vi "vi for testing code.vi"() -> ()   [LabVIEW 2020]
panel:
  out "XY Graph":T1(graph)
  out "acc 3":dbl[](array[numeric])
  out "tt 2":dbl[](array[numeric])
  out "appended path":path
  out "array":dbl[][](array[numeric])
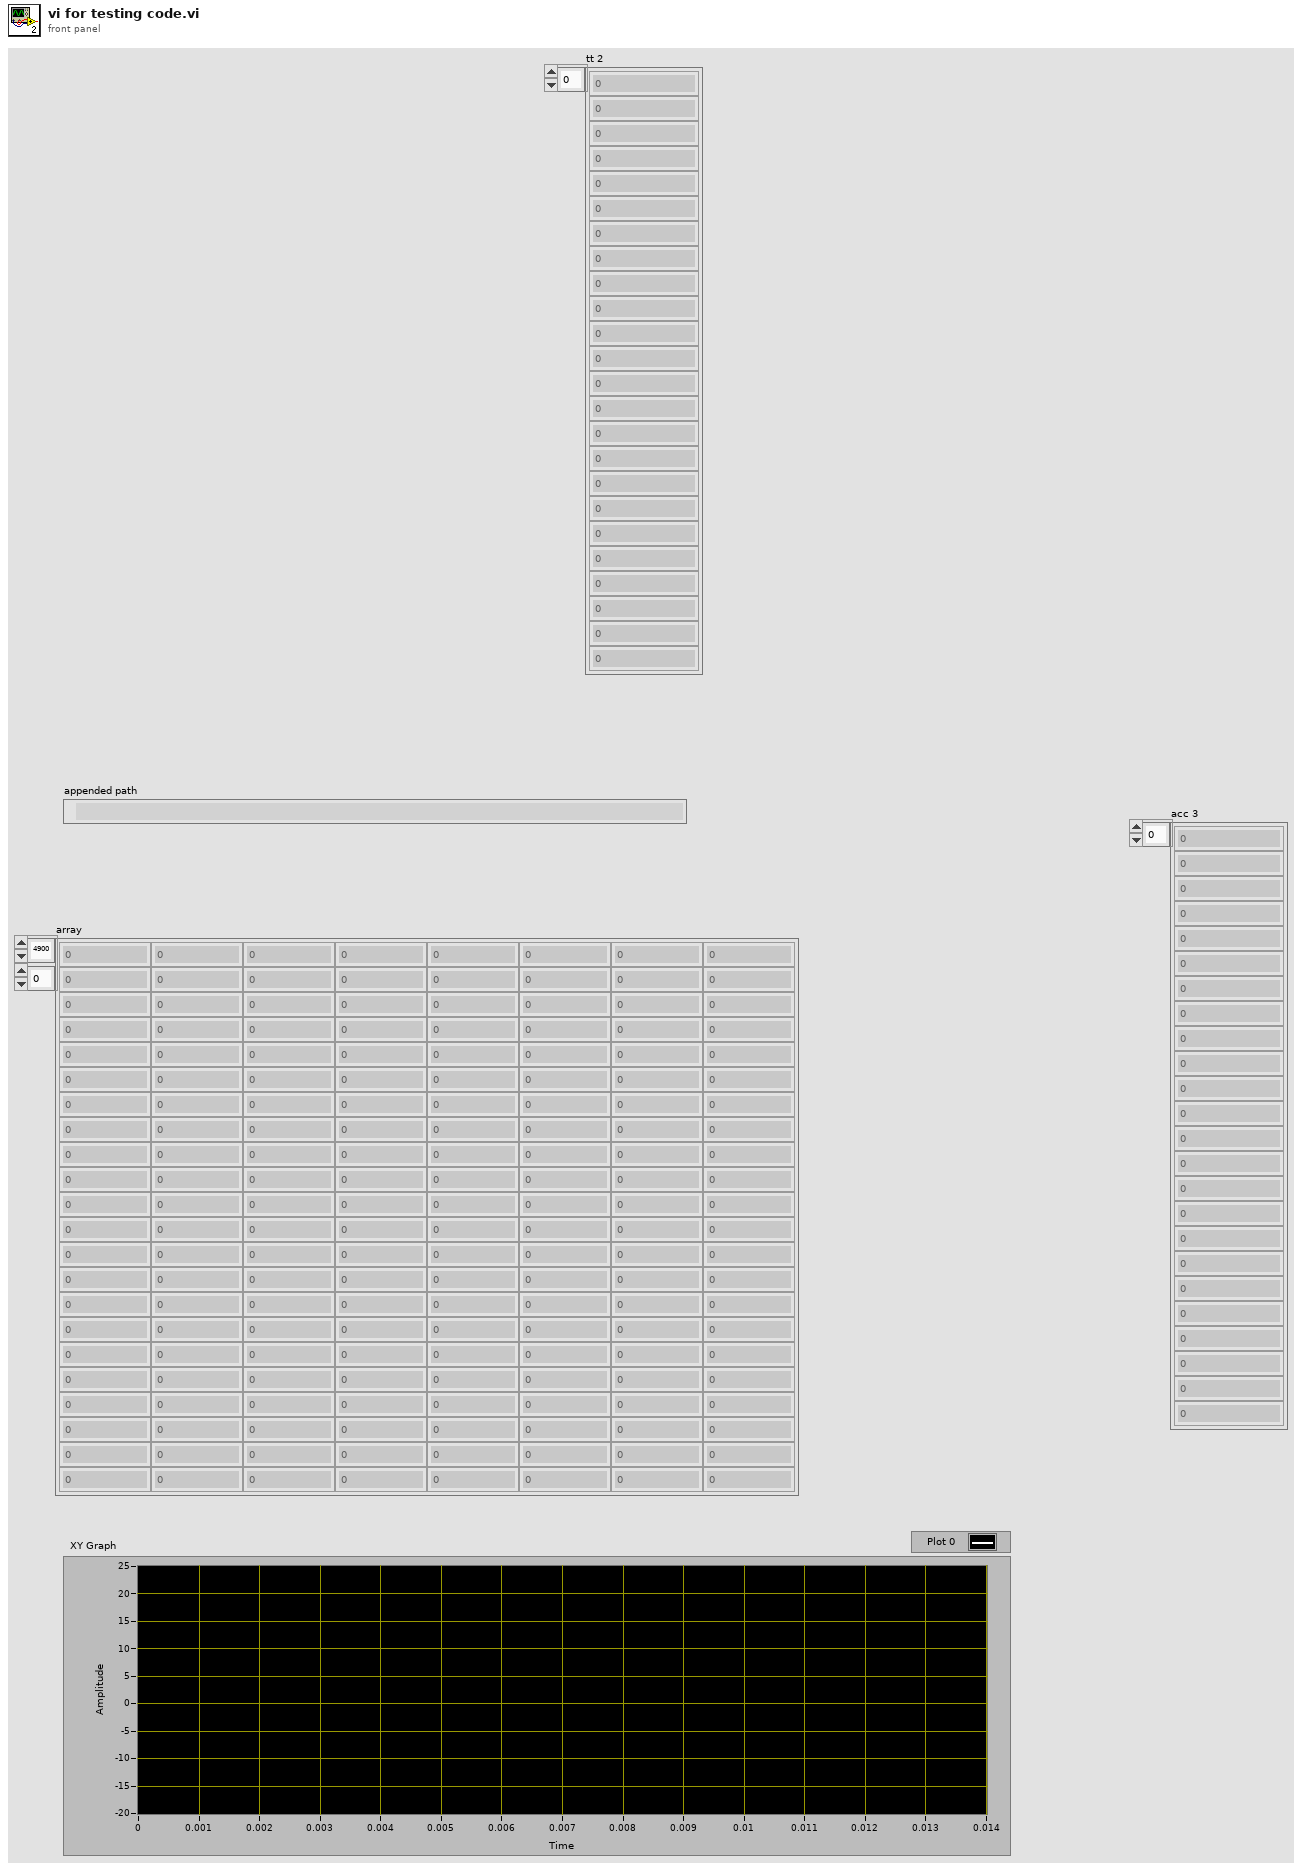
[diagram p1: front panel]
types:
  T1 = cluster{"array type (2D Dbl)":dbl[], "array type (2D Dbl)":dbl[]}
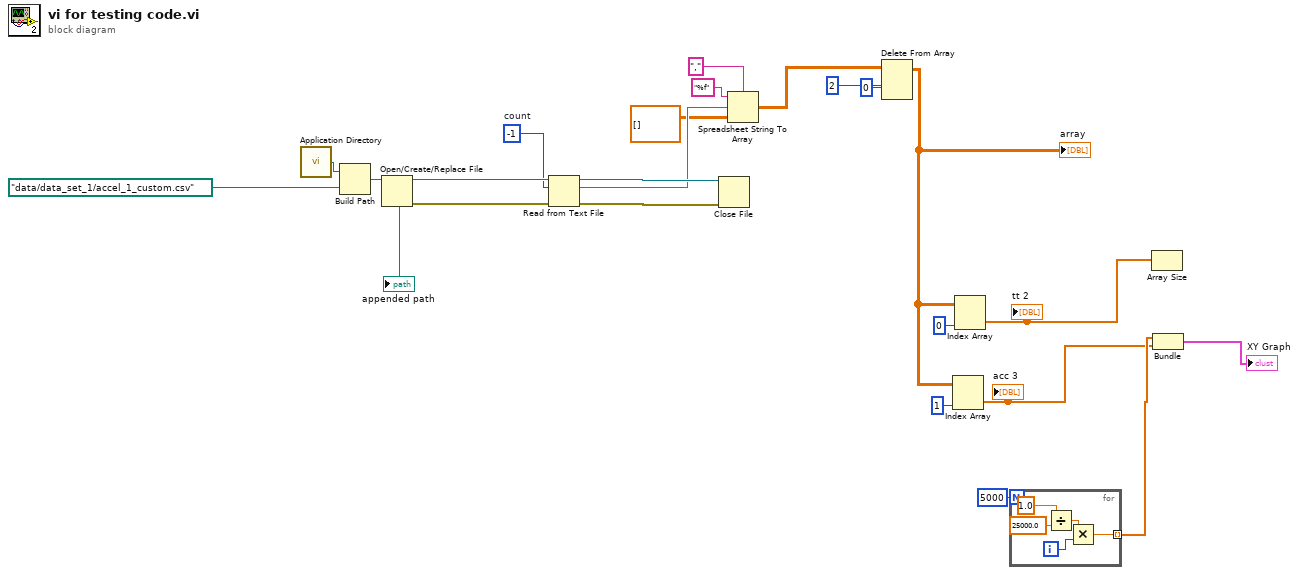
[diagram p0: block diagram]
diagram:
  w14 = -1  # count
  n1 = call <vilib>:"Application Directory.vi"() -> ("Application Directory"=w18:path)
  n2 = Build Path(base path=w18, name or relative path=path "data/data_set_1/accel_1_custom.csv" ("default name")) -> (appended path=w17:path)
  "appended path" <- w17
  n3 = Open/Create/Replace File(file path (use dialog)=w17) -> (refnum out=w22:refnum<file>, error out=w23:errorcluster)  [unwired: 5 in, 1 out]
  n4 = Read from Text File(file (use dialog)=w22, count=w14, error in=w23) -> (refnum out=w21:refnum<file>, text=w19:string, error out=w20:errorcluster)  [unwired: 1 in, 1 out]
  n5 = Close File(refnum=w21, error in=w20) -> ()  [unwired: 2 out]
  n6 = Spreadsheet String To Array(delimiter (Tab)=",", format string="%f", spreadsheet string=w19, array type (2D Dbl)=dbl[][] []) -> (array=w11:dbl[][])
  n7 = Delete From Array(array=w11, length=2, index (row)=0) -> (array with subset deleted=w6:dbl[][])  [unwired: 1 in, 1 out]
  "array" <- w6
  n8 = Index Array(array=w6, index (col)=1 ("disabled index (col)")) -> (element=w1:dbl[])  [unwired: 1 in]
  "acc 3" <- w1
  n9 = Index Array(array=w6, index (col)=0 ("disabled index (col)")) -> (element=w4:dbl[])  [unwired: 1 in]
  "tt 2" <- w4
  n10 = for {
    N: 5000 -> [_]
    tunnel: [w24] -> w2 mode=indexing
    i -> [w28]
    n11 = Divide(x=1.0, y=25000.0) -> (x/y=w25:dbl)
    n12 = Multiply(x=w25, y=w28) -> (x*y=w24:dbl)
  }
  n13 = Array Size(array=w4) -> ()  [unwired: 1 out]
  n14 = Bundle(w2, "array type (2D Dbl)"=w1) -> (→"XY Graph":cluster{dbl[], "array type (2D Dbl)":dbl[]})  [unwired: 1 in]
